vi "[ModBus Ethernet Example Slave_16].vi"() -> ()   [LabVIEW 2010]
uses:
  MB Slave Init (poly).vi
  MB Globals.vi
  MB Slave Read All Coils (poly).vi
  MB Slave Read All Holding Registers (poly).vi
  MB Slave Write Input Registers (poly).vi
  MB Slave Write Discrete Inputs (poly).vi
  <vilib>/addons/internet/NI_InternetTK_Core_VIs.lvlib
panel:
  out "本机IP":string
  in  "Discrete Inputs (Read only)":bool[](array[boolean])=[FALSE, FALSE, FALSE, FALSE, FALSE, FALSE, FALSE, FALSE, FALSE, FALSE, FALSE, FALSE, FALSE, FALSE, FALSE, FALSE, FALSE, FALSE, FALSE, FALSE, FALSE, FALSE, FALSE, FALSE, FALSE, FALSE, FALSE, FALSE, TRUE, TRUE]
  in  "Input Registers (Read Only)":u16[](array[numeric])=[0, 0, 0, 0]
  in  "TCP服务端口":u16=502
  in  "Stop":bool
  out "Holding Registers":u16[](array[numeric]) caption="Holding Registers (Master can write in these registers)"
  out "Coils":bool[](array[boolean]) caption="Coils (Master can write coils)"
  # "TCP Settings"
  # "Slave Registers"
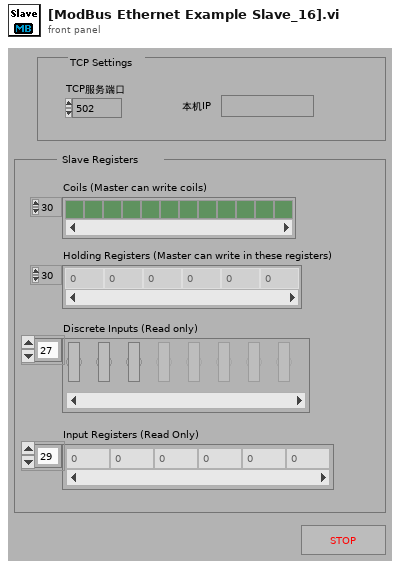
[diagram p1: front panel]
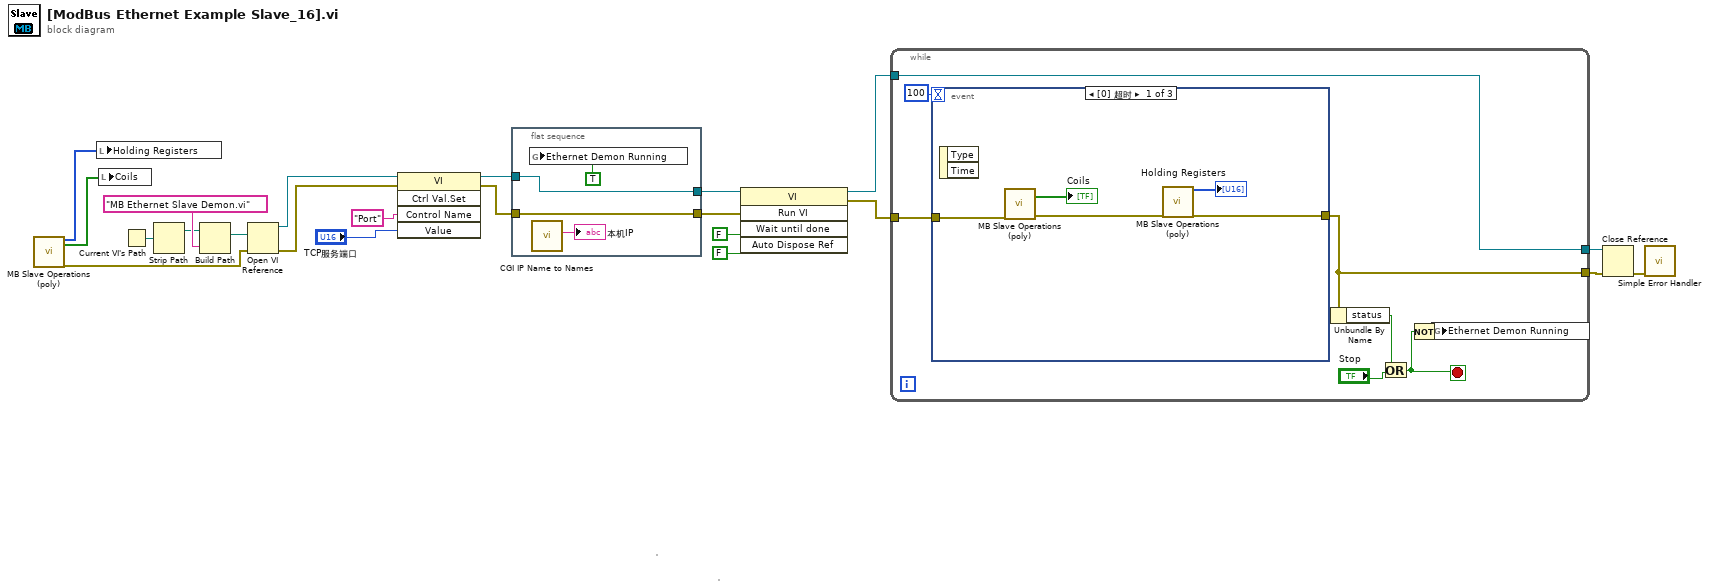
[diagram p0: block diagram]
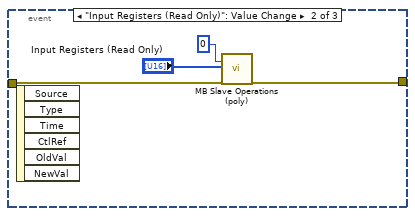
[diagram p2: hidden frame]
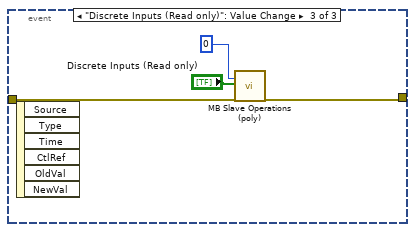
[diagram p3: hidden frame]
diagram:
  n1 = call-poly "MB Slave Operations (poly).vi"() -> ("Holding Registers"=w22:u16[], "Coils"=w6:bool[], "error out"=w9:errorcluster)  [unwired: 1 in, 16 out]
  n2 = local write "Holding Registers"(w22) -> ()
  n3 = local write "Coils"(w6) -> ()
  n4 = Current VI's Path() -> (path=w18:path)
  n5 = Strip Path(path=w18) -> (stripped path=w19:path)  [unwired: 1 out]
  n6 = Build Path(base path=w19, name or relative path="MB Ethernet Slave Demon.vi") -> (appended path=w21:path)
  n7 = Open VI Reference(vi path=w21, error in (no error)=w9) -> (vi reference=w15:refnum<vi>, error out=w14:errorcluster)  [unwired: 4 out]
  n8 = invoke class="VI" method="Ctrl Val.Set"(reference=w15, error in=w14, "Control Name"="Port", "Value"="TCP服务端口") -> (reference out=w2:refnum<vi>, error out=w3:errorcluster)  [unwired: 1 in, 3 out]
  n9 = flat-sequence {
    tunnel: [w26] -> w8
    tunnel: w3 -> [w26]
    tunnel: [w24] -> w5
    tunnel: w2 -> [w24]
    frame #0 {
      n10 = global write "MB Globals.vi" "Ethernet Demon Running"(TRUE ("Slave Demon Running")) -> ()
      n11 = call <vilib>:"CGI IP Name to Names.vi"() -> ("domain name"=→"本机IP":string)  [unwired: 6 in, 1 out]
    }
  }
  n12 = invoke class="VI" method="Run VI"(reference=w5, error in=w8, "Wait until done"=FALSE, "Auto Dispose Ref"=FALSE) -> (reference out=w11:refnum<vi>, error out=w7:errorcluster)  [unwired: 1 in, 3 out]
  n13 = while {
    tunnel: [w29] -> w12
    tunnel: w11 -> [w29]
    tunnel: [w28] -> w10
    tunnel: w7 -> [w27]
    stop <- w30 stop-if-true
    n14 = event shown="[0] 超时" {
      selector: _ -> [_ _ _]
      dyn-events: _ -> [_ _ _]
      timeout: 100 -> [_ _ _]
      tunnel: w27 -> [w39 w43 w47]
      tunnel: [w36 w41 w45] -> w28
      event Timeout {
        n15 = event-data() -> ()  [unwired: 3 out]
        n16 = call-poly "MB Slave Operations (poly).vi"("error in"=w39) -> ("Coils"=→"Coils":bool[], "error out"=w37:errorcluster)  [unwired: 17 out]
        n17 = call-poly "MB Slave Operations (poly).vi"("error in"=w37) -> ("Holding Registers"=→"Holding Registers":u16[], "error out"=w36:errorcluster)  [unwired: 17 out]
      }
      event "Input Registers (Read Only)": Value Change {
        n18 = event-data() -> ()  [unwired: 7 out]
        n19 = call-poly "MB Slave Operations (poly).vi"("Starting Address"=u16 0 ("Address"), "Input Registers"="Input Registers (Read Only)", "error in"=w43) -> ("error out"=w41:errorcluster)  [unwired: 1 in, 15 out]
      }
      event "Discrete Inputs (Read only)": Value Change {
        n20 = event-data() -> ()  [unwired: 7 out]
        n21 = call-poly "MB Slave Operations (poly).vi"("Starting Address"=u16 0, "Discrete Inputs"="Discrete Inputs (Read only)", "error in"=w47) -> ("error out"=w45:errorcluster)  [unwired: 1 in, 15 out]
      }
    }
    n22 = Unbundle By Name(w28) -> ("status"=w33:bool)
    n23 = Or(x=w33, y="Stop") -> (x .or. y?=w30:bool)
    n24 = Not(x=w30) -> (.not. x?=w31:bool)
    n25 = global write "MB Globals.vi" "Ethernet Demon Running"(w31) -> ()
  }
  n26 = Close Reference(reference=w12, error in (no error)=w10) -> (error out=w4:errorcluster)
  n27 = call <vilib>:"Simple Error Handler.vi"("error in (no error)"=w4) -> ()  [unwired: 1 in, 8 out]
